vi "Write Sessions.vi"(10 "Sessions":refnum<class "Session.lvclass">[](array[class]), 11 "ConnectionHandler in":refnum<class "ConnectionHandler.lvclass">) -> (3 "ConnectionHandler":refnum<class "ConnectionHandler.lvclass">)   [LabVIEW 2013, in "MQTT_Connection.lvlib" / "ConnectionHandler.lvclass"]
uses:
  ConnectionHandler.lvclass
  MQTT_Base/Session/Session.lvclass
  ConnectionHandler.lvclass/ConnectionHandler.ctl
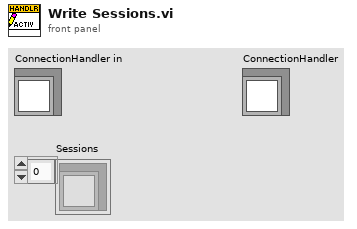
[diagram p1: front panel]
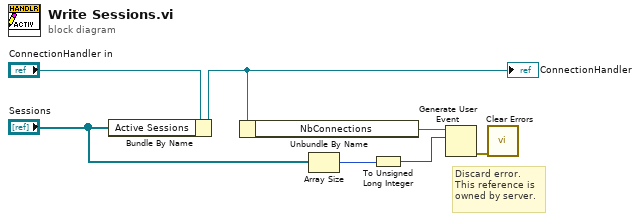
[diagram p0: block diagram]
diagram:
  # "Discard error.\nThis reference is\nowned by server."
  n1 = Bundle By Name(cluster="ConnectionHandler in", "Active Sessions"="Sessions") -> (w6:refnum<class "ConnectionHandler.lvclass">)
  "ConnectionHandler" <- w6
  n2 = Unbundle By Name(w6) -> ("NbConnections"=w5:refnum<user-event>)
  n3 = Array Size(array="Sessions") -> (size(s)=w3:i32)
  n4 = To Unsigned Long Integer(number=w3) -> (unsigned 32bit integer=w1:u32)
  n5 = Generate User Event(user event=w5, event data cluster=w1) -> (error out=w2:errorcluster)  [unwired: 2 in, 1 out]
  n6 = call <vilib>:"Clear Errors.vi"("error in (no error)"=w2) -> ()  [unwired: 6 in, 1 out]
